vi "calculate zm.vi"(0 "W_A [raw signal]":dbl format="%#_13g", 5 "W_B [raw signal]":dbl format="%#_13g", 7 "Z":T1 {"zm" format="%.8f"; "zt" format="%.8f"; "zi" format="%.8f"}, 9 "T [K]":dbl format="%#_13g", 11 "Chi_A":dbl format="%#_13g") -> (8 "Z (out)":T1 {"zm" format="%.8f"; "zt" format="%.8f"; "zi" format="%.8f"})   [LabVIEW 2010, in "LicorLI7000.lvlib"]
uses:
  LicorLI7000.lvlib
  Z parameter.ctl
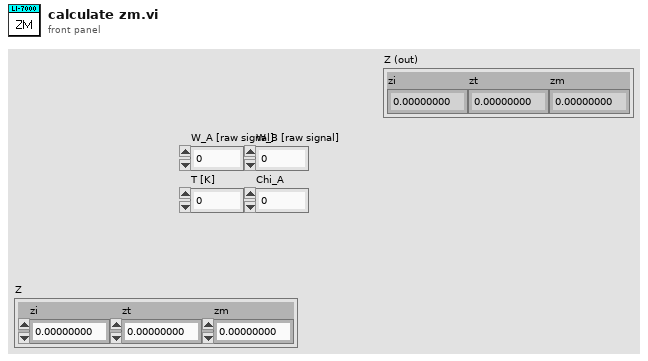
[diagram p1: front panel]
types:
  T1 = typedef "LicorLI7000.lvlib/Z parameter.ctl" = cluster{"zi":dbl, "zt":dbl, "zm":dbl}
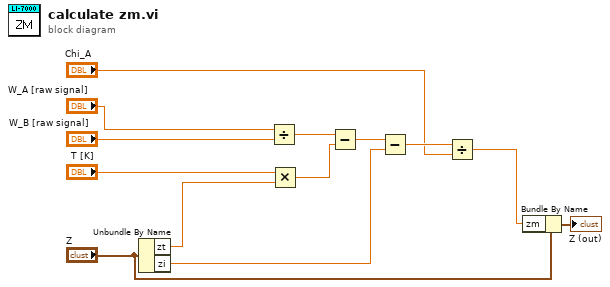
[diagram p0: block diagram]
diagram:
  n1 = Unbundle By Name("Z") -> ("zt"=w5:dbl, "zi"=w4:dbl)
  n2 = Divide(x="W_A [raw signal]", y="W_B [raw signal]") -> (x/y=w11:dbl)
  n3 = Multiply(x="T [K]", y=w5) -> (x*y=w7:dbl)
  n4 = Subtract(x=w11, y=w7) -> (x-y=w10:dbl)
  n5 = Subtract(x=w10, y=w4) -> (x-y=w9:dbl)
  n6 = Divide(x=w9, y="Chi_A") -> (x/y=w2:dbl)
  n7 = Bundle By Name(cluster="Z", "zm"=w2) -> (→"Z (out)":T1)
